vi "Create Dev Panel.vi"(10 "Ex Event Actor":refnum<class "Ex Event Actor.lvclass">, 11 "Ex Queue Actor in":refnum<class "Ex Queue Actor.lvclass">) -> (0 "error out":errorcluster, 3 "Ex Queue Actor out":refnum<class "Ex Queue Actor.lvclass">)   [LabVIEW 2021, in "Ex Queue Actor.lvlib" / "Ex Queue Actor.lvclass"]
uses:
  Ex Queue Actor.lvclass
  Ex Event Actor/Ex Event Actor/Ex Event Actor.lvclass
  C:/git/jettl/src/Actor/Event Actor/Event Actor.lvclass
  Ex Queue Actor.lvclass/Ex Queue Actor.ctl
  Actor/Event Actor/Event Actor.lvclass
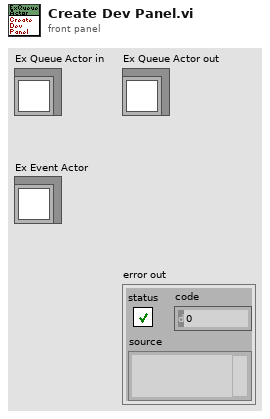
[diagram p1: front panel]
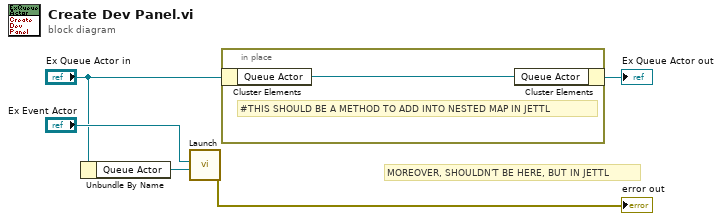
[diagram p0: block diagram]
diagram:
  # "MOREOVER, SHOULDN'T BE HERE, BUT IN JETTL"
  n1 = Unbundle By Name("Ex Queue Actor in") -> ("Queue Actor"=w4:refnum<class "Queue Actor.lvclass">)
  n2 = call "Launch.vi"("Queue Actor"=w4, "Event Actor"="Ex Event Actor") -> ("error out"=→"error out":errorcluster)  [unwired: 8 in, 1 out]
  n3 = in-place {
    # "#THIS SHOULD BE A METHOD TO ADD INTO NESTED MAP IN JETTL"
    n4 = in-place-cluster #1("Ex Queue Actor in") -> ("Queue Actor"=w6:refnum<class "Queue Actor.lvclass">)
    n5 = in-place-cluster #1("Queue Actor"=w6) -> (→"Ex Queue Actor out":refnum<class "Ex Queue Actor.lvclass">)
  }
